vi "HMI panel 2.vi"(6 "Process State":string, 8 "Elapsed time in current state":dbl format="%.2f", 9 "Sensor Data smoothed":T1 {"Sensor array"."scaled" format="%.2f"; "Sensor array"."voltage" format="%.4f"; "Time" format="%<%I:%M:%S%2u %p\n%m/%d/%Y>T"}, 10 "Current Control settings":cluster{"switch":bool, "fractional duty":dbl}[](array[cluster]) {"fractional duty" format="%#_3g"}, 11 "Set Points":T2(array[cluster])) -> ()   [LabVIEW 2010]
panel:
  out "Plant flow rate":dbl[unit](knob)
  out "Flow control valve":bool
  out "Backwash pump":bool
  out "Clearwell":dbl[unit](slide)
  # "Place this HMI panel VI in your folder and then edit this panel to make it represent your plant. I've placed a couple of examples of things you can do.\n\nHave fun!"
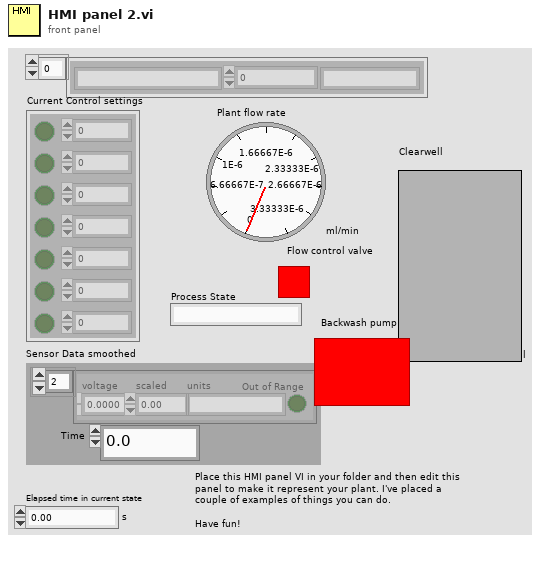
[diagram p1: front panel]
types:
  T1 = cluster{" Sensor array":cluster{"voltage":sgl, "scaled":sgl, "units":string, "Out of Range":bool}[], "Time":dbl}
  T2 = cluster{"name":string, "unit":string, "value":dbl}[]
  T3 = cluster{"name":string, "unit":string, "value":dbl}
  T4 = cluster{"voltage":sgl, "scaled":sgl, "units":string, "Out of Range":bool}[]
  T5 = cluster{"voltage":sgl, "scaled":sgl, "units":string, "Out of Range":bool}
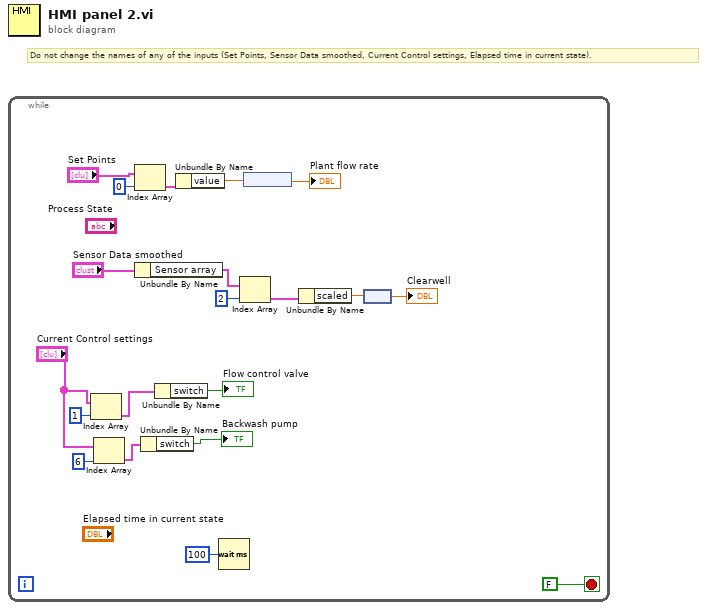
[diagram p0: block diagram]
diagram:
  # "Do not change the names of any of the inputs (Set Points, Sensor Data smoothed, Current Control settings, Elapsed time in current state)."
  n1 = while {
    stop <- FALSE stop-if-true
    n2 = Index Array(array="Current Control settings", index=1) -> (element=w11:cluster{"switch":bool, "fractional duty":dbl})
    n3 = Index Array(array="Current Control settings", index=6) -> (element=w7:cluster{"switch":bool, "fractional duty":dbl})
    n4 = Index Array(array="Set Points", index=0) -> (element=w14:T3)
    n5 = Unbundle By Name("Sensor Data smoothed") -> ("Sensor array"=w4:T4)
    n6 = Unbundle By Name(w7) -> ("switch"=→"Backwash pump":bool)
    n7 = Unbundle By Name(w11) -> ("switch"=→"Flow control valve":bool)
    n8 = Unbundle By Name(w14) -> ("value"=w13:dbl)
    n9 = Wait (ms)(milliseconds to wait=u32 100) -> ()  [unwired: 1 out]
    n10 = Index Array(array=w4, index=u32 2 ("Sensor index")) -> (element=w2:T5)
    n11 = node(w13) -> (→"Plant flow rate":dbl[unit])
    n12 = Unbundle By Name(w2) -> ("scaled"=w1:sgl)
    n13 = node(w1) -> (→"Clearwell":sgl[unit])
  }
